vi "GageMultipleRecord.vi"() -> ()   [LabVIEW 2015]
panel:
  in  "Segment":u32=1 min=1 max=5
  out "Board":string
  in  "Number Of Records":u32=100
  out "1st segment TS":string
  out "Time Interval Graph":cluster{i32[], dbl[]}(graph)
  out "Tick Frequency, Hz":u32
  in  "Run":bool=TRUE
  in  "Trigger":T1={"Slope"=0, "Level"=0, "Source"=0, "External Range"=2000, "External Coupling"=0, "External"=FALSE, "Disable"=FALSE, "External Impedance"=1} {"External Impedance" items=["50 Ohm", "HiZ"]; "External Coupling" items=["DC", "AC"]; "External Range" min=2000 max=10000 step=8000; "Slope" items=["Rising", "Falling"]; "Level" min=-100 max=100; "Source" min=0 max=64 step=1}
  in  "Reset":bool
  in  "Counter source":bool
  out "Array":dbl[](array[numeric]) format="%.2f"
  out "Status":string
  in  "Channels":T2(array[cluster])=[{"Coupling"=0, "Differential Input"=FALSE, "Direct-to-ADC"=FALSE, "Range"=2000, "Impedance"=50, "DC Offset"=0, "Filter"=0}] {"Impedance" min=50 max=1000000 step=999950; "Coupling" items=["DC", "AC"]}
  in  "Acquisition":T3={"Sample Rate"=100000000.0, "Mode"=0, "Depth"=8192.0, "Segment Size"=8192.0, "Trigger Timeout"=1000000.0, "Trigger Holdoff"=0.0, "Trigger Delay"=0.0, "Clock mode"=enum."Internal"} {"Segment Size" min=256.0 step=128.0; "Trigger Delay" min=0.0 step=128.0; "Trigger Holdoff" min=0.0 step=128.0; "Depth" min=256.0 step=128.0; "Mode" items=["Single", "Dual", "Quad", "Octal"]}
  in  "Stop":bool
  in  "Length":dbl=512.0 step=128.0
  in  "Start Point":dbl step=1.0
  out "Waveform Graph":cluster{dbl, dbl, "Data in Volts":dbl[][]}(graph) caption="Record 1  of  5"
  # "Time stamp"
  # "of"
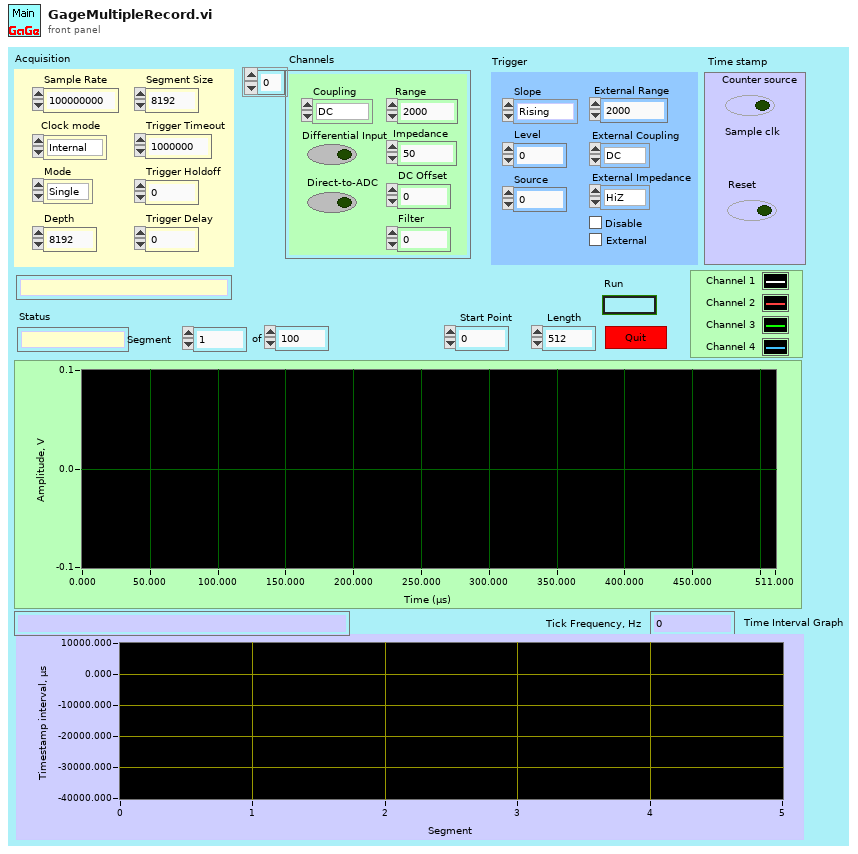
[diagram p1: front panel]
types:
  T1 = cluster{"Slope":u16, "Level":i32, "Source":i32, "External Range":u32, "External Coupling":u16, "External":bool, "Disable":bool, "External Impedance":u16}
  T2 = cluster{"Coupling":u16, "Differential Input":bool, "Direct-to-ADC":bool, "Range":u32, "Impedance":u32, "DC Offset":i32, "Filter":i32}[]
  T3 = cluster{"Sample Rate":dbl, "Mode":u16, "Depth":dbl, "Segment Size":dbl, "Trigger Timeout":dbl, "Trigger Holdoff":dbl, "Trigger Delay":dbl, "Clock mode":enum16{"Internal", "External", "Reference"}}
  T4 = cluster{"Handle":u32, "Sample size":u32, "Resolution":i32, "Offset":i32, "Channels":u32, "Boards":u32}
  T5 = cluster{"Coupling":u16, "Differential Input":bool, "Direct-to-ADC":bool, "Range":u32, "Impedance":u32, "DC Offset":i32, "Filter":i32}
  T6 = cluster{string, "Differential Input":bool, "Direct-to-ADC":bool, "Range":u32, "Impedance":u32, "DC Offset":i32, u32}
  T7 = cluster{"RingText.Text":string, "Level":i32, "Source":i32, "External Range":u32, "RingText.Text":string, "External":bool, "Disable":bool, "RingText.Text":string}
  T8 = cluster{"RingText.Text":string, "Level":i32, "Source":i32, "External Range":u32, "RingText.Text":string, "External":bool, "Disable":bool, "RingText.Text":string}[]
  T9 = cluster{"Sample Rate":dbl, "Clock mode":enum16{"Internal", "External", "Reference"}, "RingText.Text":string, "Depth":dbl, "Segment Size":dbl, "Trigger Timeout":dbl, "Trigger Holdoff":dbl, "Trigger Delay":dbl}
  T10 = cluster{"Handle":u32, "Sample Size":u32, "Resolution":i32, "Offset":i32, "Channels":u32, "Boards":u32}
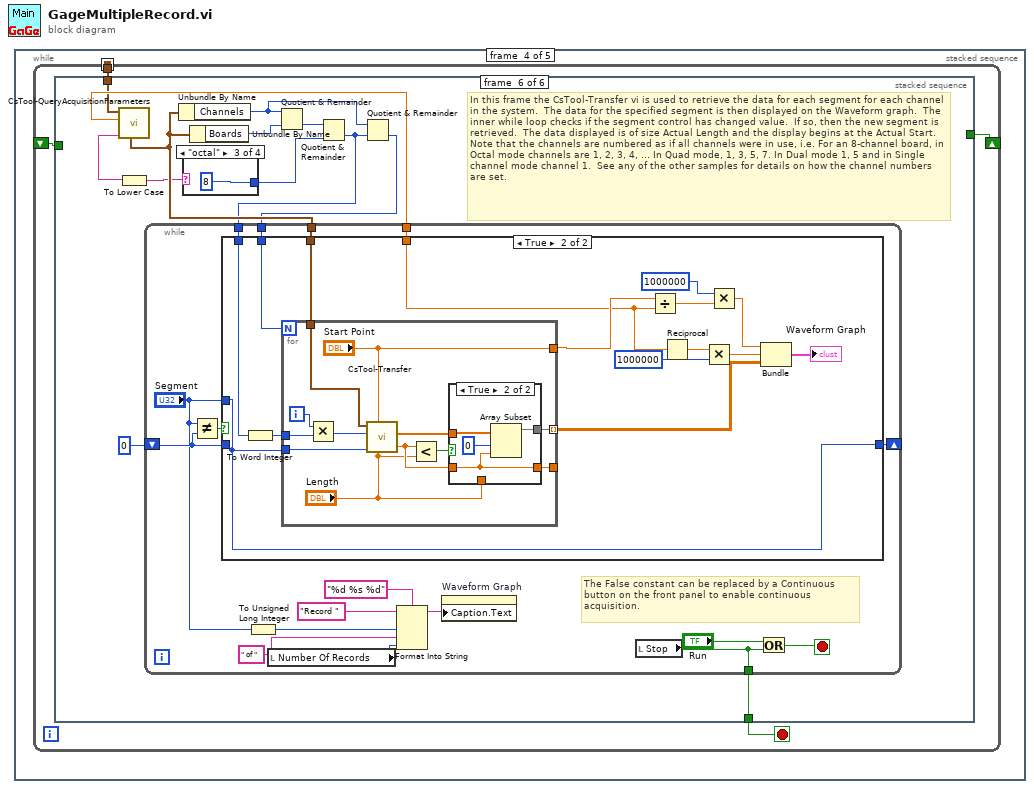
[diagram p0: block diagram]
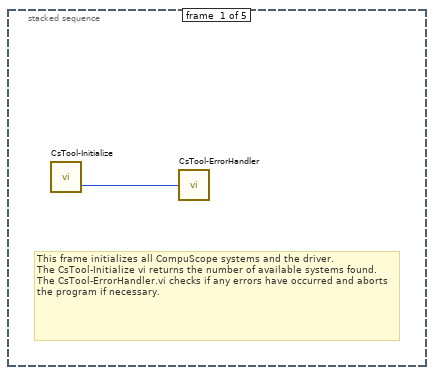
[diagram p2: hidden frame]
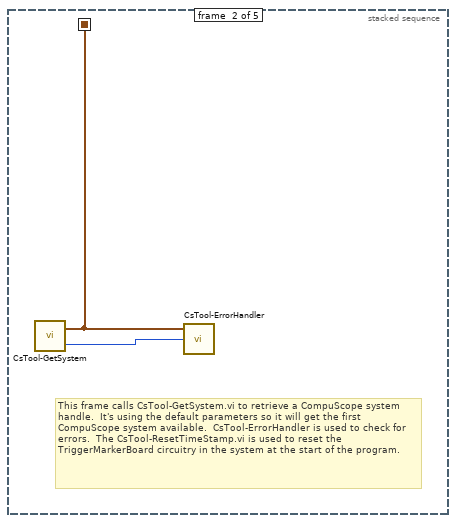
[diagram p3: hidden frame]
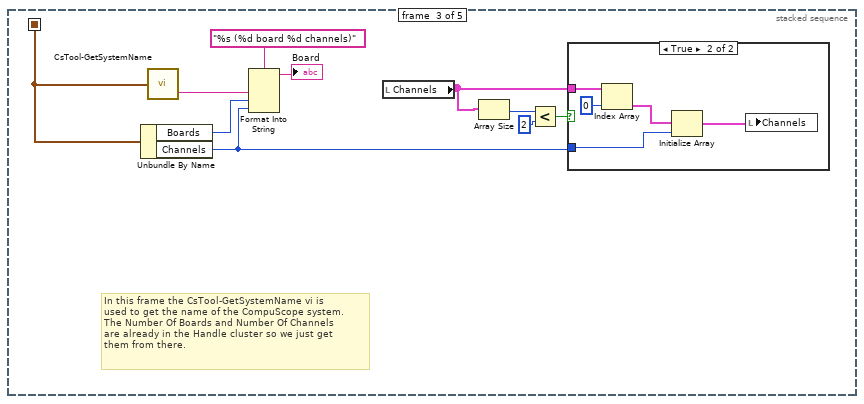
[diagram p4: hidden frame]
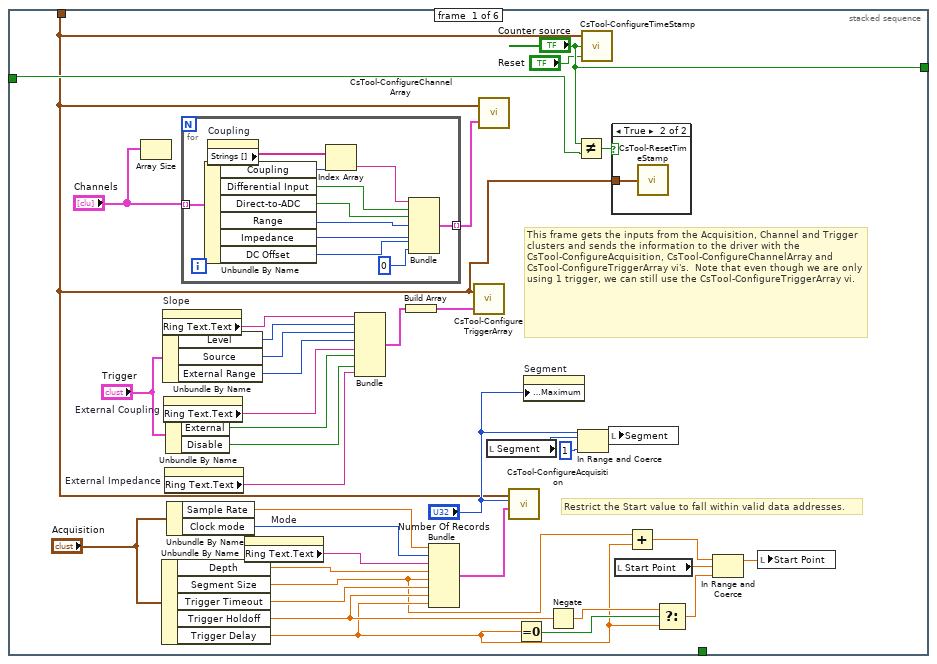
[diagram p6: hidden frame]
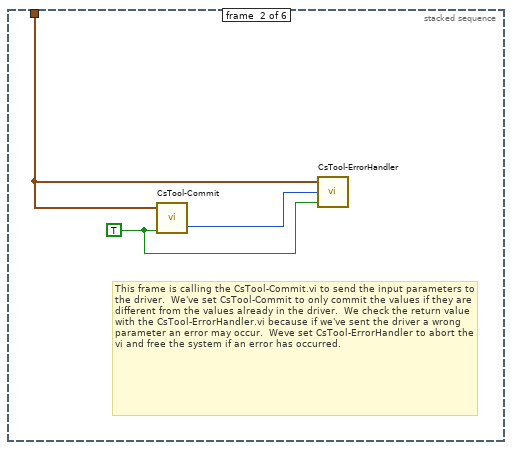
[diagram p8: hidden frame]
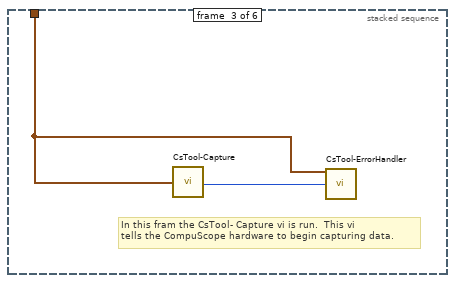
[diagram p9: hidden frame]
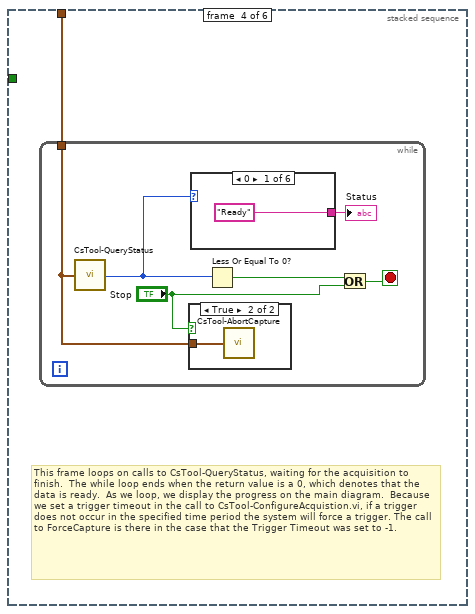
[diagram p10: hidden frame]
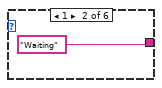
[diagram p12: hidden frame]
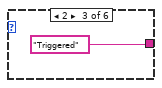
[diagram p13: hidden frame]
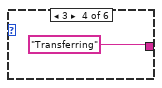
[diagram p14: hidden frame]
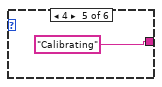
[diagram p15: hidden frame]
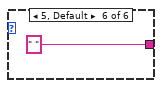
[diagram p16: hidden frame]
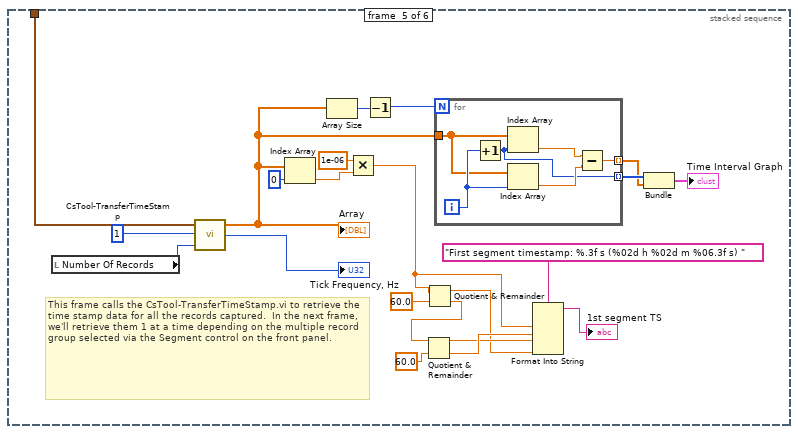
[diagram p17: hidden frame]
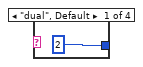
[diagram p18: hidden frame]
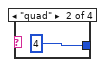
[diagram p19: hidden frame]
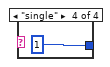
[diagram p20: hidden frame]
diagram:
  n1 = stacked-sequence {
    seq-local: [_ w2 _ _ _] -> [_ _ w13 w19 w190]
    frame #0 {
      # "This frame initializes all CompuScope systems and the driver.\nThe CsTool-Initialize vi returns the number of available systems found.  The CsTool-ErrorHandler.vi checks if any errors have occurred and aborts the program if necessary."
      n2 = call <userlib>:"CsTool-Initialize.vi"() -> ("Error Code"=w1:i32)  [unwired: 1 out]
      n3 = call <userlib>:"CsTool-ErrorHandler.vi"("Error Code"=w1) -> ()  [unwired: 2 in, 1 out]
    }
    frame #1 {
      # "This frame calls CsTool-GetSystem.vi to retrieve a CompuScope system handle.  It's using the default parameters so it will get the first CompuScope system available.  CsTool-ErrorHandler is used to check for errors.  The CsTool-ResetTimeStamp.vi is used to reset the TriggerMarkerBoard circuitry in the system at the start of the program."
      n4 = call <userlib>:"CsTool-GetSystem.vi"() -> ("Error Code"=w3:i32, "Handle Cluster"=w2:T4)  [unwired: 4 in]
      n5 = call <userlib>:"CsTool-ErrorHandler.vi"("Error Code"=w3, "Handle Cluster"=w2) -> ()  [unwired: 1 in, 1 out]
    }
    frame #2 {
      # "In this frame the CsTool-GetSystemName vi is \nused to get the name of the CompuScope system.\nThe Number Of Boards and Number Of Channels \nare already in the Handle cluster so we just get \nthem from there."
      n6 = Unbundle By Name(w13) -> ("Boards"=w5:u32, "Channels"=w6:u32)
      n7 = call <userlib>:"CsTool-GetSystemName.vi"("Handle Cluster"=w13) -> ("System Name"=w7:string)  [unwired: 1 out]
      n8 = Format Into String(format string="%s (%d board %d channels)", w7, w5, w6) -> (resulting string=→"Board":string)  [unwired: 2 in, 1 out]
      n9 = local read "Channels"() -> (w11:T2)
      n10 = Array Size(array=w11) -> (size(s)=w10:i32)
      n11 = Less?(x=w10, y=2) -> (x < y?=w12:bool)
      n12 = case shown="True" w12 {
        tunnel: w6 -> [_ w18]
        tunnel: w11 -> [_ w16]
        frame False {
        }
        frame True {
          n13 = Index Array(array=w16, index=0) -> (element=w15:T5)
          n14 = Initialize Array(w15, w18) -> (w14:T2)
          n15 = local write "Channels"(w14) -> ()
        }
      }
    }
    frame #3 {
      n16 = while {
        tunnel: w19 -> [w22]
        shift-right: [w21] -> _
        shift-left: _ -> [w20]
        stop <- w23 stop-if-true
        n17 = stacked-sequence {
          tunnel: w22 -> [w33 w74 w77 w79 w114 w130]
          tunnel: [_ _ _ _ _ w132] -> w23
          tunnel: ["Counter source" _ _ _ _ _] -> w21
          tunnel: w20 -> [w36 _ _ _ _ _]
          frame #0 {
            # "Restrict the Start value to fall within valid data addresses."
            # "This frame gets the inputs from the Acquisition, Channel and Trigger clusters and sends the information to the driver with the CsTool-ConfigureAcquisition, CsTool-ConfigureChannelArray and CsTool-ConfigureTriggerArray vi's.  Note that even though we are only using 1 trigger, we can still use the CsTool-ConfigureTriggerArray vi."
            n18 = Array Size(array="Channels") -> ()  [unwired: 1 out]
            n19 = Unbundle By Name("Acquisition") -> ("Depth"=w57:dbl, "Segment Size"=w26:dbl, "Trigger Timeout"=w59:dbl, "Trigger Holdoff"=w31:dbl, "Trigger Delay"=w27:dbl)
            n20 = property on="Slope" class="Ring (strict)"() -> ("Ring Text.Text"=w47:string)  [unwired: 2 in, 2 out]
            n21 = Unbundle By Name("Trigger") -> ("Level"=w49:i32, "Source"=w51:i32, "External Range"=w52:u32)
            n22 = property on="External Coupling" class="Ring (strict)"() -> ("Ring Text.Text"=w46:string)  [unwired: 2 in, 2 out]
            n23 = property on="External Impedance" class="Ring (strict)"() -> ("Ring Text.Text"=w45:string)  [unwired: 2 in, 2 out]
            n24 = Unbundle By Name("Trigger") -> ("External"=w50:bool, "Disable"=w53:bool)
            n25 = Unbundle By Name("Acquisition") -> ("Sample Rate"=w56:dbl, "Clock mode"=w58:enum16{"Internal", "External", "Reference"})
            n26 = for {
              tunnel: "Channels" -> [w71] mode=indexing
              tunnel: [w72] -> w60 mode=indexing
              n27 = Unbundle By Name(w71) -> ("Coupling"=w67:u16, "Differential Input"=w73:bool, "Direct-to-ADC"=w66:bool, "Range"=w65:u32, "Impedance"=w64:u32, "DC Offset"=w63:i32)
              n28 = property on="Coupling" class="Ring (strict)"() -> ("Strings []"=w70:string[])  [unwired: 2 in, 2 out]
              n29 = Index Array(array=w70, index=w67) -> (element=w69:string)
              n30 = Bundle(w69, "Differential Input"=w73, "Direct-to-ADC"=w66, "Range"=w65, "Impedance"=w64, "DC Offset"=w63, u32 0) -> (w72:T6)  [unwired: 1 in]
            }
            n31 = property on="Mode" class="Ring (strict)"() -> ("Ring Text.Text"=w55:string)  [unwired: 2 in, 2 out]
            n32 = Bundle("RingText.Text"=w47, "Level"=w49, "Source"=w51, "External Range"=w52, "RingText.Text"=w46, "External"=w50, "Disable"=w53, "RingText.Text"=w45) -> (w44:T7)  [unwired: 1 in]
            n33 = Build Array(w44) -> (w43:T8)
            n34 = Bundle("Sample Rate"=w56, "Clock mode"=w58, "RingText.Text"=w55, "Depth"=w57, "Segment Size"=w26, "Trigger Timeout"=w59, "Trigger Holdoff"=w31, "Trigger Delay"=w27) -> (w42:T9)  [unwired: 1 in]
            n35 = call <userlib>:"CsTool-ConfigureTriggerArray.vi"("Triggers"=w43, "Handle Cluster"=w33) -> ()  [unwired: 1 out]
            n36 = call <userlib>:"CsTool-ConfigureChannelArray.vi"("Channels"=w60, "Handle Cluster"=w33) -> ()  [unwired: 1 out]
            n37 = local read "Segment"() -> (w38:u32)
            n38 = call <userlib>:"CsTool-ConfigureAcquisition.vi"("Handle Cluster"=w33, "Segment Count (1)"="Number Of Records", "Acquisition"=w42) -> ()  [unwired: 2 in, 1 out]
            n39 = Equal To 0?(x=w27) -> (x = 0?=w30:bool)
            n40 = property on="Segment" class="DigNum (strict)"("Data Entry Limits:Maximum"="Number Of Records") -> ()  [unwired: 2 in, 2 out]
            n41 = Negate(x=w31) -> (-x=w29:dbl)
            n42 = Not Equal?(x="Counter source", y=w36) -> (x != y?=w37:bool)
            n43 = In Range and Coerce(upper limit="Number Of Records", x=w38, lower limit=u32 1) -> (coerced(x)=w41:u32)  [unwired: 1 out]
            n44 = call <userlib>:"CsTool-ConfigureTimeStamp.vi"("Reset"="Reset", "Sample Clock"="Counter source", "Handle Cluster"=w33) -> ()  [unwired: 1 out]
            n45 = local write "Segment"(w41) -> ()
            n46 = case shown="True" w37 {
              tunnel: w33 -> [_ w62]
              frame False {
              }
              frame True {
                n47 = call <userlib>:"CsTool-ResetTimeStamp.vi"("Handle Cluster"=w62) -> ()  [unwired: 1 out]
              }
            }
            n48 = local read "Start Point"() -> (w32:dbl)
            n49 = Add(x=w26, y=w27) -> (x+y=w25:dbl)
            n50 = Select(t=w29, s=w30, f=w27) -> (s? t:f=w28:dbl)
            n51 = In Range and Coerce(upper limit=w25, x=w32, lower limit=w28) -> (coerced(x)=w24:dbl)  [unwired: 1 out]
            n52 = local write "Start Point"(w24) -> ()
          }
          frame #1 {
            w75 = TRUE
            # "This frame is calling the CsTool-Commit.vi to send the input parameters to the driver.  We've set CsTool-Commit to only commit the values if they are different from the values already in the driver.  We check the return value with the CsTool-ErrorHandler.vi because if we've sent the driver a wrong parameter an error may occur.  Weve set CsTool-ErrorHandler to abort the vi and free the system if an error has occurred."
            n53 = call <userlib>:"CsTool-Commit.vi"("OnlyOnChange (t)"=w75, "Handle Cluster"=w74) -> ("Error Code"=w76:i32)  [unwired: 1 in, 1 out]
            n54 = call <userlib>:"CsTool-ErrorHandler.vi"("StopOnError (true)"=w75, "Error Code"=w76, "Handle Cluster"=w74) -> ()  [unwired: 1 out]
          }
          frame #2 {
            # "In this fram the CsTool- Capture vi is run.  This vi\ntells the CompuScope hardware to begin capturing data."
            n55 = call <userlib>:"CsTool-Capture.vi"("Handle Cluster"=w77) -> ("Error Code"=w78:i32)
            n56 = call <userlib>:"CsTool-ErrorHandler.vi"("Error Code"=w78, "Handle Cluster"=w77) -> ()  [unwired: 1 in, 1 out]
          }
          frame #3 {
            # "This frame loops on calls to CsTool-QueryStatus, waiting for the acquisition to finish.  The while loop ends when the return value is a 0, which denotes that the data is ready.  As we loop, we display the progress on the main diagram.  Because we set a trigger timeout in the call to CsTool-ConfigureAcquistion.vi, if a trigger does not occur in the specified time period the system will force a trigger. The call to ForceCapture is there in the case that the Trigger Timeout was set to -1."
            n57 = while {
              tunnel: w79 -> [w81]
              stop <- w83 stop-if-true
              n58 = call <userlib>:"CsTool-QueryStatus.vi"("Handle Cluster"=w81) -> ("Status"=w82:i32)
              n59 = case shown="True" "Stop" {
                tunnel: w81 -> [_ w86]
                frame False {
                }
                frame True {
                  n60 = call <userlib>:"CsTool-AbortCapture.vi"("Handle Cluster"=w86) -> ()  [unwired: 1 out]
                }
              }
              n61 = case shown="0" w82 {
                tunnel: ["Ready" "Waiting" "Triggered" "Transferring" "Calibrating" " "] -> w85
                frame 0 {
                }
                frame 1 {
                }
                frame 2 {
                }
                frame 3 {
                }
                frame 4 {
                }
                frame 5, Default {
                }
              }
              "Status" <- w85
              n62 = Less Or Equal To 0?(x=w82) -> (x <= 0?=w84:bool)
              n63 = Or(x=w84, y="Stop") -> (x .or. y?=w83:bool)
            }
          }
          frame #4 {
            # "This frame calls the CsTool-TransferTimeStamp.vi to retrieve the time stamp data for all the records captured.  In the next frame, we'll retrieve them 1 at a time depending on the multiple record group selected via the Segment control on the front panel."
            n64 = local read "Number Of Records"() -> (w112:u32)
            n65 = call <userlib>:"CsTool-TransferTimeStamp.vi"("Length (1)"=w112, "Segment (1)"=1, "Handle Cluster"=w114) -> ("Tick Frequency"=→"Tick Frequency, Hz":u32, "TS Time"=w108:dbl[])  [unwired: 1 out]
            "Array" <- w108
            n66 = Index Array(array=w108, index=0) -> (element=w106:dbl)
            n67 = Array Size(array=w108) -> (size(s)=w110:i32)
            n68 = Multiply(x=1e-06, y=w106) -> (x*y=w100:dbl)
            n69 = Decrement(x=w110) -> (x-1=w109:i32)
            n70 = Quotient & Remainder(x=w100, y=60.0) -> (x-y*floor(x/y)=w97:dbl, floor(x/y)=w103:dbl)
            n71 = Quotient & Remainder(x=w103, y=60.0) -> (x-y*floor(x/y)=w98:dbl, floor(x/y)=w99:dbl)
            n72 = for {
              N: w109 -> [_]
              tunnel: w108 -> [w117]
              tunnel: [w116] -> w94 mode=indexing
              tunnel: [w115] -> w95 mode=indexing
              i -> [w120]
              n73 = Increment(x=w120) -> (x+1=w115:i32)
              n74 = Index Array(array=w117, index=w115) -> (element=w119:dbl)
              n75 = Index Array(array=w117, index=w120) -> (element=w118:dbl)
              n76 = Subtract(x=w119, y=w118) -> (x-y=w116:dbl)
            }
            n77 = Format Into String(format string="First segment timestamp: %.3f s (%02d h %02d m %06.3f s) ", w100, w99, w98, w97) -> (resulting string=→"1st segment TS":string)  [unwired: 2 in, 1 out]
            n78 = Bundle(w95, w94) -> (→"Time Interval Graph":cluster{i32[], dbl[]})  [unwired: 1 in]
          }
          frame #5 {
            # "In this frame the CsTool-Transfer vi is used to retrieve the data for each segment for each channel in the system.  The data for the specified segment is then displayed on the Waveform graph.  The inner while loop checks if the segment control has changed value.  If so, then the new segment is retrieved.  The data displayed is of size Actual Length and the display begins at the Actual Start. Note that the channels are numbered as if all channels were in use, i.e. For an 8-channel board, in Octal mode channels are 1, 2, 3, 4, ... In Quad mode, 1, 3, 5, 7. In Dual mode 1, 5 and in Single channel mode channel 1.  See any of the other samples for details on how the channel numbers are set."
            n79 = call <userlib>:"CsTool-QueryAcquisitionParameters.vi"("Handle Cluster"=w130) -> ("Output Handle Cluster"=w129:T10, "Mode"=w128:string, "Sample Rate"=w131:dbl)  [unwired: 8 out]
            n80 = To Lower Case(string=w128) -> (all lower case string=w127:string)
            n81 = Unbundle By Name(w129) -> ("Channels"=w123:u32)
            n82 = case shown="\"octal\"" w127 {
              tunnel: [2 4 8 1] -> w124
              frame "dual", Default {
              }
              frame "quad" {
              }
              frame "octal" {
              }
              frame "single" {
              }
            }
            n83 = Unbundle By Name(w129) -> ("Boards"=w126:u32)
            n84 = Quotient & Remainder(x=w123, y=w126) -> (floor(x/y)=w125:u32)  [unwired: 1 out]
            n85 = Quotient & Remainder(x=w125, y=w124) -> (floor(x/y)=w122:u32)  [unwired: 1 out]
            n86 = Quotient & Remainder(x=w123, y=w122) -> (floor(x/y)=w121:u32)  [unwired: 1 out]
            n87 = while {
              shift-right: [w153] -> _
              shift-left: u32 0 -> [w152]
              tunnel: [w139] -> w132
              tunnel: w129 -> [w150]
              tunnel: w131 -> [w142]
              tunnel: w121 -> [w141]
              tunnel: w122 -> [w140]
              stop <- w151 stop-if-true
              # "The False constant can be replaced by a Continuous\nbutton on the front panel to enable continuous\nacquisition."
              n88 = Not Equal?(x="Segment", y=w152) -> (x != y?=w154:bool)
              n89 = case shown="True" w154 {
                tunnel: "Segment" -> [_ w163]
                tunnel: [w155 w163] -> w153
                tunnel: w152 -> [w155 _]
                tunnel: w150 -> [_ w170]
                tunnel: w142 -> [_ w167]
                tunnel: w141 -> [_ w166]
                tunnel: w140 -> [_ w165]
                frame False {
                }
                frame True {
                  n90 = To Word Integer(number=w165) -> (16bit integer=w164:i16)
                  n91 = for {
                    N: w166 -> [_]
                    tunnel: [w179] -> w169 mode=indexing
                    tunnel: w163 -> [w182]
                    tunnel: w170 -> [w178]
                    tunnel: ["Start Point"] -> w168
                    tunnel: w164 -> [w176]
                    tunnel: [w173] -> _
                    i -> [w177]
                    n92 = Multiply(x=w177, y=w176) -> (x*y=w171:i32)
                    n93 = call <userlib>:"CsTool-Transfer.vi"("Length (4096)"="Length", "Start (0)"="Start Point", "Segment (1)"=w182, "Channel (0)"=w171, "Handle Cluster"=w178) -> ("Actual Length"=w175:dbl, "Data in Volts"=w180:dbl[])  [unwired: 1 in, 2 out]
                    n94 = Less?(x=w175, y="Length") -> (x < y?=w181:bool)
                    n95 = case shown="True" w181 {
                      tunnel: w180 -> [w184 w188]
                      tunnel: [w184 w186] -> w179
                      tunnel: w175 -> [_ w185]
                      tunnel: [w183 w185] -> w173
                      tunnel: "Length" -> [w183 _]
                      frame False {
                      }
                      frame True {
                        n96 = Array Subset(array=w188, index=0, length=w185) -> (w186:dbl[])
                      }
                    }
                  }
                  n97 = Divide(x=w168, y=w167) -> (x/y=w157:dbl)
                  n98 = Reciprocal(x=w167) -> (1/x=w158:dbl)
                  n99 = Multiply(x=w158, y=1000000) -> (x*y=w161:dbl)
                  n100 = Multiply(x=1000000, y=w157) -> (x*y=w160:dbl)
                  n101 = Bundle(w160, w161, "Data in Volts"=w169) -> (→"Waveform Graph":cluster{dbl, dbl, "Data in Volts":dbl[][]})  [unwired: 1 in]
                }
              }
              n102 = To Unsigned Long Integer(number="Segment") -> (unsigned 32bit integer=w148:u32)
              n103 = local read "Number Of Records"() -> (w146:u32)
              n104 = Format Into String(format string="%d %s %d", initial string="Record ", w148, " of ", w146) -> (resulting string=w145:string)  [unwired: 1 in, 1 out]
              n105 = property on="Waveform Graph" class="WFGraph (strict)"("Caption.Text"=w145) -> ()  [unwired: 2 in, 2 out]
              n106 = local read "Stop"() -> (w139:bool)
              n107 = Or(x="Run", y=w139) -> (x .or. y?=w151:bool)
            }
          }
        }
      }
    }
    frame #4 {
      # "We set the Stop button (actually it's local variable) to False here so when the vi stops the Stop button will not stay depressed."
      # "In this frame, which is reached when the Stop\nis pressed, the CompuScope system is freed by\nrunning the CsTool-FreeSystem vi.  This frees any resources\nused by the system and makes it available for another\nprogram to use."
      n108 = local write "Stop"(FALSE) -> ()
      n109 = call <userlib>:"CsTool-FreeSystem.vi"("Handle Cluster"=w190) -> ()  [unwired: 1 out]
    }
  }
